vi "I2C_tester.vi"() -> ()   [LabVIEW 2018]
uses:
  <vilib>/myRIO/Instrument Drivers/Onboard IO/I2C/typedefs/I2C User Configuration.ctl
  <vilib>/myRIO/Instrument Drivers/Onboard IO/I2C/typedefs/I2C Transfer Rate.ctl
  <vilib>/myRIO/Instrument Drivers/Onboard IO/I2C/typedefs/I2C Reference.ctl
  <vilib>/myRIO/Common/Instrument Driver Framework/Utilities/typedefs/myRIO Generic Hardware Reference.ctl
  <vilib>/myRIO/Common/Instrument Driver Framework/Utilities/typedefs/Hardware Version Enum.ctl
  <vilib>/myRIO/Common/Instrument Driver Framework/Utilities/typedefs/myRIO v1.0 Reference.ctl
  <vilib>/myRIO/Common/Instrument Driver Framework/Utilities/typedefs/Generic FPGA Reference.ctl
  <vilib>/myRIO/Common/Instrument Driver Framework/myRIO v1.0/I2C/typedefs/I2C Channels Enum.ctl
  <vilib>/myRIO/Instrument Drivers/Onboard IO/I2C/typedefs/I2C Configuration.ctl
  <vilib>/userdefined/High Color/nirio_resource_hc.ctl
  <vilib>/myRIO/Common/Instrument Driver Framework/Utilities/vis/Is FPGA Ref Available.vi
  <vilib>/myRIO/Common/Instrument Driver Framework/myRIO v1.0/I2C/vis/myRIO v1.1 Open I2C.vi
  <vilib>/myRIO/Instrument Drivers/Onboard IO/I2C/vis/Configure.vi
  <vilib>/myRIO/Instrument Drivers/Onboard IO/I2C/vis/Write Read.vi
  <vilib>/myRIO/Instrument Drivers/Onboard IO/I2C/vis/Write.vi
  <vilib>/myRIO/Common/Instrument Driver Framework/Utilities/vis/Validate Channels.vi
  <vilib>/myRIO/Common/Instrument Driver Framework/myRIO v1.0/I2C/vis/myRIO v1.0 Reserve I2C.vi
  <vilib>/myRIO/Common/Instrument Driver Framework/myRIO v1.0/I2C/vis/myRIO v1.0 Build MUX Configuration I2C.vi
  <vilib>/myRIO/Common/Instrument Driver Framework/myRIO v1.0/Resource Manager/vis/myRIO v1.0 Reserve Channel List.vi
  <vilib>/myRIO/Common/Instrument Driver Framework/myRIO v1.0/Resource Manager/vis/myRIO v1.0 Create Configuration List.vi
  <vilib>/myRIO/Common/Instrument Driver Framework/myRIO v1.0/Resource Manager/vis/myRIO v1.0 Reserve Channel.vi
  <vilib>/myRIO/Common/Instrument Driver Framework/myRIO v1.0/Resource Manager/vis/myRIO v1.0 Unreserve Channel.vi
  <vilib>/myRIO/Common/Instrument Driver Framework/myRIO v1.0/Resource Manager/vis/myRIO v1.0 Build Mutex Name.vi
  <vilib>/Utility/VariantDataType/GetNumericInfo.vi
  <vilib>/Utility/error.llb/Error Cluster From Error Code.vi
  <vilib>/myRIO/Common/Instrument Driver Framework/myRIO v1.0/myRIO v1.1 Open.vi
  <vilib>/myRIO/Common/Instrument Driver Framework/Utilities/vis/IO Manager.vi
  <vilib>/myRIO/Common/Instrument Driver Framework/Utilities/vis/Configuration Manager.vi
  <vilib>/myRIO/Common/Instrument Driver Framework/myRIO v1.0/Resource Manager/vis/myRIO v1.0 Configure IO.vi
  <vilib>/myRIO/Common/Instrument Driver Framework/myRIO v1.0/myRIO v1.0 Close.vi
  <vilib>/myRIO/Common/Instrument Driver Framework/myRIO v1.0/I2C/vis/myRIO v1.0 Configure I2C.vi
  <vilib>/myRIO/Common/Instrument Driver Framework/myRIO v1.0/I2C/vis/myRIO v1.0 Write I2C.vi
  <vilib>/myRIO/Common/Instrument Driver Framework/myRIO v1.0/I2C/vis/myRIO v1.0 Read I2C.vi
  <vilib>/myRIO/Express VI/Onboard IO/I2C/I2C Express VI.xnode
  <vilib>/myRIO/Instrument Drivers/Onboard IO/I2C/vis/myRIO I2C Open.xnode
  <vilib>/myRIO/Instrument Drivers/Onboard IO/I2C/I2C.lvlib
panel:
  in  "Register (Lux)":T1(ring)
  out "register":u8 format="%02x"
  in  "Register (RGB)":T2(ring)
  in  "Gain":enum8{"1x", "4x", "16x", "60x"}(ring)
  out "Data":u16
  out "Bytes Read":u8[](array[numeric])
  out "Not connected":bool
  in  "Stop Button":bool
  # "RGB"
  # "Not available on the lux sensor yet"
  # "Lux"
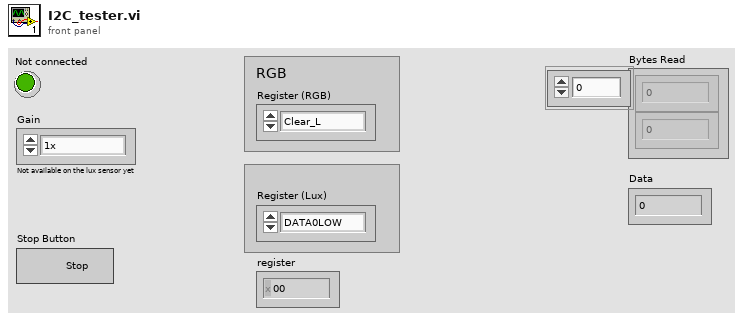
[diagram p1: front panel]
types:
  T1 = enum16{"DATA0LOW", "DATA0HIGH", "DATA1LOW", "DATA1HIGH"}
  T2 = enum8{"Clear_L", "Clear_H", "Red_L", "Red_H", "Green_L", "Green_H", "Blue_L", "Blue_H"}
  T3 = typedef "I2C.lvlib/I2C Reference.ctl" = cluster{"myRIO Reference":T4, "I2C Channels Enum":T8, "I2C Configuration":T9}
  T4 = typedef "myRIO Generic Hardware Reference.ctl" = cluster{"myRIO Model":T5, "myRIO Hardware Reference":T6}
  T5 = typedef "Hardware Version Enum.ctl" = enum16{"Unknown", "myRIO-1900", "myRIO-1950", "roboRIO", "NI ELVIS RIO CM", "ELVIS III"}
  T6 = typedef "myRIO v1.0 Reference.ctl" = cluster{"Generic FPGA Reference":T7, "Allow multiple opens":bool}
  T7 = typedef "Generic FPGA Reference.ctl" = refnum<k20>
  T8 = typedef "I2C Channels Enum.ctl" = enum16{"Not Connected", "A/I2C", "B/I2C", "I2C/I2C"}
  T9 = typedef "I2C.lvlib/I2C Configuration.ctl" = cluster{"I2C Transfer Rate":T10}
  T10 = typedef "I2C.lvlib/I2C Transfer Rate.ctl" = enum16{"Standard mode (100 kbps)", "Fast mode (400 kbps)"}
  T11 = typedef "I2C.lvlib/I2C User Configuration.ctl" = cluster{"I2C Transfer Rate":T10}
  T12 = typedef "nirio_resource_hc.ctl" = tag
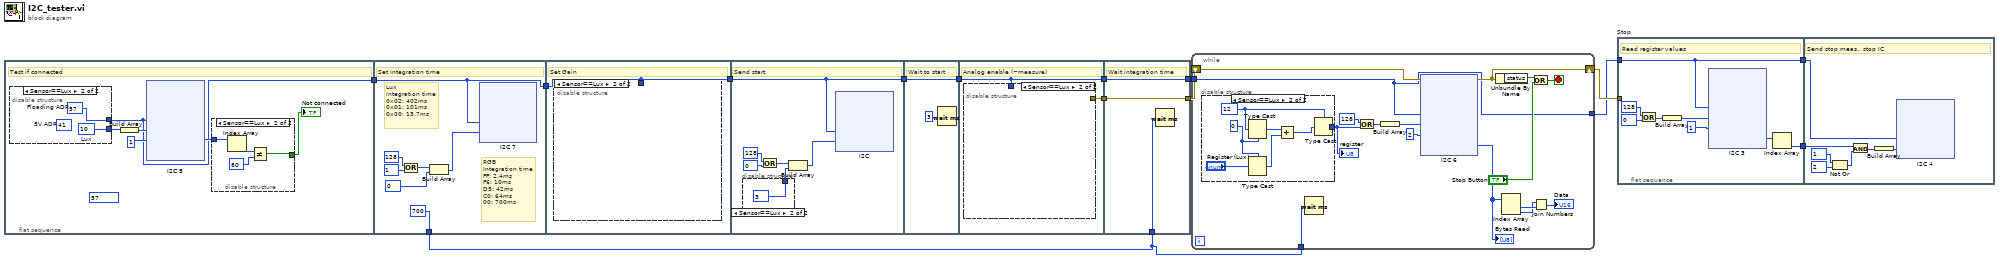
[diagram p0: block diagram]
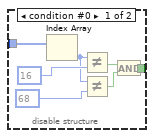
[diagram p2: hidden frame]
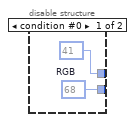
[diagram p3: hidden frame]
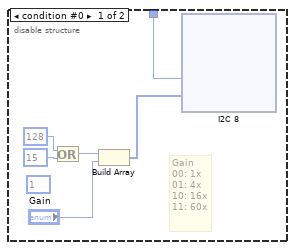
[diagram p4: hidden frame]
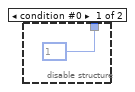
[diagram p5: hidden frame]
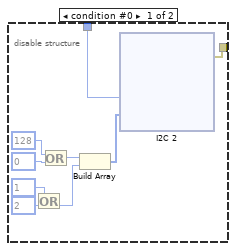
[diagram p6: hidden frame]
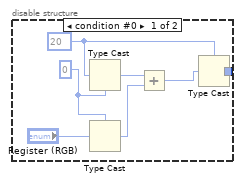
[diagram p7: hidden frame]
diagram:
  n1 = flat-sequence {
    tunnel: [w15] -> w9
    tunnel: [u32 700] -> w10
    tunnel: w9 -> [w76]
    tunnel: [w76] -> w7
    tunnel: [w121] -> w8
    tunnel: w7 -> [w121]
    tunnel: w8 -> [w166]
    tunnel: [w166] -> w6
    tunnel: w6 -> [w212]
    tunnel: [w212] -> w5
    tunnel: [w215] -> w13
    tunnel: w5 -> [w214]
    tunnel: [w214] -> w4
    tunnel: [w265] -> w12
    tunnel: w13 -> [w265]
    tunnel: w10 -> [w264]
    tunnel: w4 -> [w263]
    tunnel: [w263] -> w3
    frame #0 {
      (unwired) u8 57 ("Slave Address (7-bit)")
      # "Test if connected"
      n2 = disable-structure shown="Sensor==Lux" {
        disable-tunnel: [w33 w35] -> w16
        disable-tunnel: [u8 41 ("Slave Address (7-bit)") w34] -> w15
        frame condition #0 {
          w33 = u8 68  # RGB
        }
        frame condition #1 (active) {
          (unwired) u8 41  # 5V ADR
          w34 = u8 57  # Floading ADR
          w35 = u8 10  # Lux
        }
      }
      n3 = Build Array(w16) -> (w17:u8[])
      n4 = xnode "I2C 5"("Slave Address (7-bit)"=w15, "Bytes to Write"=w17, "Byte Count"=u32 1) -> ("Bytes Read"=w20:u8[])  [unwired: 1 in, 1 out]
      n5 = disable-structure shown="Sensor==Lux" {
        disable-tunnel: w20 -> [w27 w31]
        disable-tunnel: [w21 w28] -> w19
        frame condition #0 {
          n6 = Index Array(array=w27) -> (element=w25:u8)  [unwired: 1 in]
          n7 = Not Equal?(x=w25, y=u8 16 ("Slave Address (7-bit)")) -> (x != y?=w23:bool)
          n8 = Not Equal?(x=w25, y=u8 68 ("Slave Address (7-bit)")) -> (x != y?=w22:bool)
          n9 = And(x=w23, y=w22) -> (x .and. y?=w21:bool)
        }
        frame condition #1 (active) {
          n10 = Index Array(array=w31) -> (element=w30:u8)  [unwired: 1 in]
          n11 = Not Equal?(x=w30, y=u8 80 ("Slave Address (7-bit)")) -> (x != y?=w28:bool)
        }
      }
      "Not connected" <- w19
    }
    frame #1 {
      # "Lux\nIntegration time\n0x02: 402ms\n0x01: 101ms\n0x00: 13.7ms"
      # "RGB\nIntegration time\nFF: 2.4ms\nF6: 10ms\nD5: 42ms\nC0: 64ms\n00: 700ms"
      # "Set Integration time"
      n12 = Or(x=u8 128 ("Slave Address (7-bit)"), y=u8 1 ("Slave Address (7-bit)")) -> (x .or. y?=w80:u8)
      n13 = Build Array(w80, u8 0 ("Slave Address (7-bit)")) -> (w81:u8[])
      n14 = xnode "I2C 7"("Slave Address (7-bit)"=w76, "Bytes to Write"=w81) -> ()  [unwired: 1 in, 1 out]
    }
    frame #2 {
      # "Set Gain"
      n15 = disable-structure shown="Sensor==Lux" {
        disable-tunnel: w121 -> [w122 _]
        frame condition #0 {
          (unwired) u8 1 ("Slave Address (7-bit)")
          # "Gain\n00: 1x\n01: 4x\n10: 16x\n11: 60x"
          n16 = Or(x=u8 128 ("Slave Address (7-bit)"), y=u8 15 ("Slave Address (7-bit)")) -> (x .or. y?=w125:u8)
          n17 = Build Array(w125, "Gain") -> (w124:u8[])
          n18 = xnode "I2C 8"("Slave Address (7-bit)"=w122, "Bytes to Write"=w124) -> ()  [unwired: 1 in, 1 out]
        }
        frame condition #1 (active) {
        }
      }
    }
    frame #3 {
      # "Send start"
      n19 = disable-structure shown="Sensor==Lux" {
        disable-tunnel: [u8 1 ("Slave Address (7-bit)") u8 3 ("Slave Address (7-bit)")] -> w167
        frame condition #0 {
        }
        frame condition #1 (active) {
        }
      }
      n20 = Or(x=u8 128 ("Slave Address (7-bit)"), y=u8 0 ("Slave Address (7-bit)")) -> (x .or. y?=w169:u8)
      n21 = Build Array(w169, w167) -> (w168:u8[])
      n22 = xnode "I2C"("Slave Address (7-bit)"=w166, "Bytes to Write"=w168) -> ()  [unwired: 1 in, 1 out]
    }
    frame #4 {
      # "Wait to start"
      n23 = Wait (ms)(milliseconds to wait=u32 3) -> ()  [unwired: 1 out]
    }
    frame #5 {
      # "Analog enable (~measure)"
      n24 = disable-structure shown="Sensor==Lux" {
        disable-tunnel: [w217 _] -> w215
        disable-tunnel: w214 -> [w216 _]
        frame condition #0 {
          n25 = Or(x=u8 1 ("Slave Address (7-bit)"), y=u8 2 ("Slave Address (7-bit)")) -> (x .or. y?=w219:u8)
          n26 = Or(x=u8 128 ("Slave Address (7-bit)"), y=u8 0 ("Slave Address (7-bit)")) -> (x .or. y?=w223:u8)
          n27 = Build Array(w223, w219) -> (w220:u8[])
          n28 = xnode "I2C 2"("Slave Address (7-bit)"=w216, "Bytes to Write"=w220) -> ("error out"=w217:errorcluster)  [unwired: 1 in]
        }
        frame condition #1 (active) {
        }
      }
    }
    frame #6 {
      # "Wait integration time"
      n29 = Wait (ms)(milliseconds to wait=w264) -> ()  [unwired: 1 out]
    }
  }
  n30 = while {
    shift-right: [w275] -> w11
    shift-left: w12 -> [w276]
    tunnel: w10 -> [w267]
    tunnel: w3 -> [w266]
    tunnel: [w266] -> w2
    stop <- w274 stop-if-true
    n31 = disable-structure shown="Sensor==Lux" {
      disable-tunnel: [w287 w294] -> w268
      frame condition #0 {
        w283 = u16 0
        w284 = u8 20 ("Slave Address (7-bit)")
        n32 = Type Cast(type=w283, x=w284) -> (*(type *) &x=w282:u16)
        n33 = Type Cast(type=w283, x="Register (RGB)") -> (*(type *) &x=w285:u16)
        n34 = Add(x=w282, y=w285) -> (x+y=w288:u16)
        n35 = Type Cast(type=w284, x=w288) -> (*(type *) &x=w287:u8)
      }
      frame condition #1 (active) {
        w291 = u16 0
        w292 = u8 12 ("Slave Address (7-bit)")
        n36 = Type Cast(type=w291, x=w292) -> (*(type *) &x=w290:u16)
        n37 = Type Cast(type=w291, x="Register (Lux)") -> (*(type *) &x=w293:u16)
        n38 = Add(x=w290, y=w293) -> (x+y=w295:u16)
        n39 = Type Cast(type=w292, x=w295) -> (*(type *) &x=w294:u8)
      }
    }
    "register" <- w268
    n40 = Wait (ms)(milliseconds to wait=w267) -> ()  [unwired: 1 out]
    n41 = Or(x=u8 128 ("Slave Address (7-bit)"), y=w268) -> (x .or. y?=w278:u8)
    n42 = Build Array(w278) -> (w279:u8[])
    n43 = xnode "I2C 6"("Slave Address (7-bit)"=w266, "Bytes to Write"=w279, "Byte Count"=u32 2, "error in (no error)"=w276) -> ("Bytes Read"=w272:u8[], "error out"=w275:errorcluster)
    "Bytes Read" <- w272
    n44 = Unbundle By Name(w275) -> ("status"=w273:bool)
    n45 = Index Array(array=w272) -> (element #1=w271:u8, element #2=w270:u8)  [unwired: 2 in]
    n46 = Or(x=w273, y="Stop Button") -> (x .or. y?=w274:bool)
    n47 = Join Numbers(hi=w270, lo=w271) -> ((hi.lo)=→"Data":u16)
  }
  n48 = flat-sequence "Stop" {
    tunnel: [w337] -> w14
    tunnel: w11 -> [_]
    tunnel: w2 -> [w336]
    tunnel: [w336] -> w1
    tunnel: w14 -> [w387]
    tunnel: w1 -> [w384]
    frame #0 {
      # "Read register values"
      n49 = Or(x=u8 128 ("Slave Address (7-bit)"), y=u8 0 ("Slave Address (7-bit)")) -> (x .or. y?=w342:u8)
      n50 = Build Array(w342) -> (w340:u8[])
      n51 = xnode "I2C 3"("Slave Address (7-bit)"=w336, "Bytes to Write"=w340, "Byte Count"=u32 1) -> ("Bytes Read"=w338:u8[])  [unwired: 1 in, 1 out]
      n52 = Index Array(array=w338) -> (element=w337:u8)  [unwired: 1 in]
    }
    frame #1 {
      # "Send stop meas., stop IC"
      n53 = Not Or(1:u8 2 ("Slave Address (7-bit)"), 2:u8 1 ("Slave Address (7-bit)")) -> (0:w388:u8)
      n54 = And(x=w387, y=w388) -> (x .and. y?=w386:u8)
      n55 = Build Array(w386) -> (w385:u8[])
      n56 = xnode "I2C 4"("Slave Address (7-bit)"=w384, "Bytes to Write"=w385) -> ()  [unwired: 1 in, 1 out]
    }
  }
